vi "Hardware triggered acquisition - polling.vi"() -> ()   [LabVIEW 2015]
uses:
  SubVIs/Parameters Get & Set/Get Parameters/Get NumberOfQueuedFrames.vi
  SubVIs/Parameters Get & Set/Set Parameters/Set ExposureTime_us.vi
  SubVIs/Parameters Get & Set/Set Parameters/Set FramesPerTrigger_zeroForUnlimited.vi
  SubVIs/Parameters Get & Set/Set Parameters/Set OperationMode.vi
  C:/code/Host/Installer/Scientific Camera Interfaces/LabVIEW/64_bit/Library_X64/Thorlabs.TSI.TLCameraInterfaces.dll
  64_bit/Library_X64/Thorlabs.TSI.TLCameraInterfaces.dll
  SubVIs/Parameters Get & Set/Set Parameters/Set Gain.vi
panel:
  in  "Gain":u32 max=1023
  in  "Exposure (ms)":u32=100
  in  "stop":bool
  out "Intensity Graph":u16[][](graph)
  out "FrameNumber":u32
  in  "Frames Per Trigger":u32=1
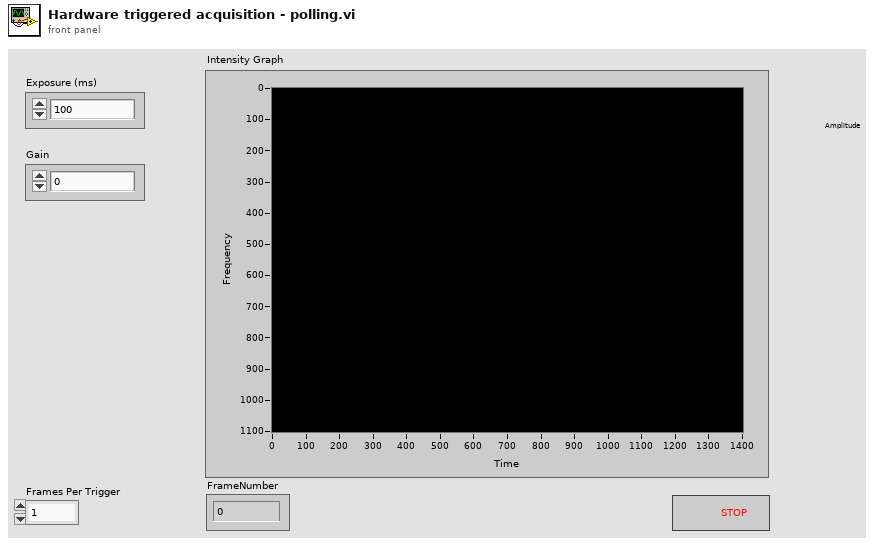
[diagram p1: front panel]
types:
  T1 = enum8{"Enabled", "Disabled", "Disabled and Grayed Out"}
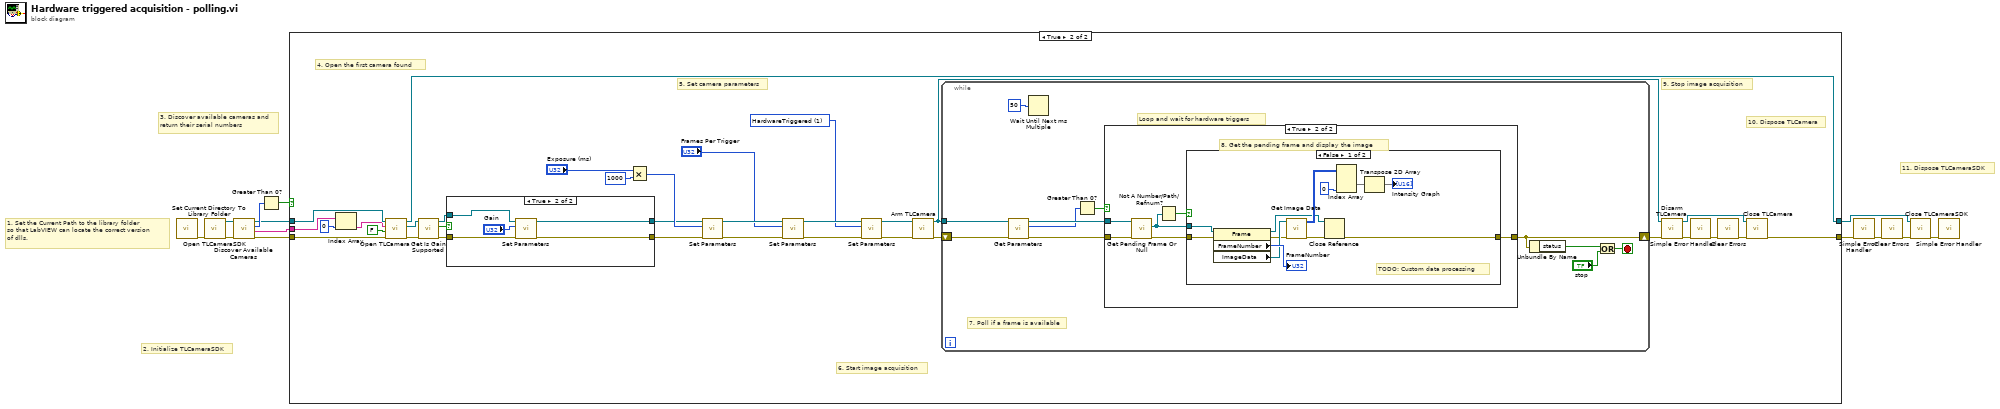
[diagram p0: block diagram]
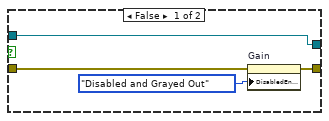
[diagram p3: hidden frame]
diagram:
  # "1. Set the Current Path to the library folder\nso that LabVIEW can locate the correct version\nof dlls."
  # "11. Dispose TLCameraSDK"
  # "3. Discover available cameras and\nreturn their serial numbers"
  # "2. Initialize TLCameraSDK"
  n1 = call "Set Current Directory To Library Folder.vi"() -> ("error out"=w7:errorcluster)  [unwired: 11 in]
  n2 = call "Open TLCameraSDK.vi"("error in (no error)"=w7) -> ("error out"=w6:errorcluster, "Thorlabs.TSI.TLCameraInterfaces.ITLCameraSDK"=w5:refnum<k24>)  [unwired: 9 in]
  n3 = call "Discover Available Cameras.vi"("error in (no error)"=w6, "Thorlabs.TSI.TLCameraInterfaces.ITLCameraSDK"=w5) -> ("error out"=w9:errorcluster, "Serial Numbers"=w11:string[], "Number of Cameras"=w13:i32, "Thorlabs.TSI.TLCameraInterfaces.ITLCameraSDK"=w10:refnum<k24>)  [unwired: 6 in]
  n4 = Greater Than 0?(x=w13) -> (x > 0?=w12:bool)
  n5 = case shown="True" w12 {
    tunnel: w11 -> [_ w47]
    tunnel: w10 -> [w14 w48]
    tunnel: w9 -> [w15 w38]
    tunnel: [w15 w35] -> w2
    tunnel: [w14 w43] -> w8
    frame False {
    }
    frame True {
      w23 = 1 items=["SoftwareTriggered", "HardwareTriggered", "Bulb", "Reserved1", "Reserved2"] ("OperationMode")
      # "10. Dispose TLCamera"
      # "9. Stop image acquisition"
      # "6. Start image acquisition"
      # "5. Set camera parameters"
      # "4. Open the first camera found"
      n6 = Index Array(array=w47, index=0) -> (element=w37:string)
      n7 = call "Open TLCamera.vi"("error in (no error)"=w38, "isDiagnosticsMessagesEnabled"=FALSE, "Camera serial number"=w37, "Thorlabs.TSI.TLCameraInterfaces.ITLCameraSDK"=w48) -> ("error out"=w19:errorcluster, "Thorlabs.TSI.TLCameraInterfaces.ITLCamera"=w18:refnum<k24>, "Thorlabs.TSI.TLCameraInterfaces.ITLCameraSDK"=w43:refnum<k24>)  [unwired: 5 in]
      n8 = call "Get Is Gain Supported.vi"("error in (no error)"=w19, "Thorlabs.TSI.TLCameraInterfaces.ITLCamera"=w18) -> ("error out"=w20:errorcluster, "Is Gain Supported?"=w22:bool, "Thorlabs.TSI.TLCameraInterfaces.ITLCamera"=w21:refnum<k24>)  [unwired: 7 in]
      n9 = case shown="True" w22 {
        tunnel: w21 -> [w50 w55]
        tunnel: w20 -> [w49 w57]
        tunnel: [w51 w56] -> w16
        tunnel: [w50 w54] -> w17
        frame False {
          n10 = property on="Gain" class="DigNum (strict)"(error in=w49, "DisabledEnum"=T1."Disabled and Grayed Out" ("Disabled")) -> (error out=w51:errorcluster)  [unwired: 1 in, 1 out]
        }
        frame True {
          n11 = call-poly "Set Parameters.vi"("error in (no error)"=w57, "Gain"="Gain", "Thorlabs.TSI.TLCameraInterfaces.ITLCamera"=w55) -> ("error out"=w56:errorcluster, "Thorlabs.TSI.TLCameraInterfaces.ITLCamera"=w54:refnum<k24>)  [unwired: 7 in]
        }
      }
      n12 = Multiply(x="Exposure (ms)", y=u32 1000) -> (x*y=w25:u32)
      n13 = call-poly "Set Parameters.vi"("error in (no error)"=w16, "ExposureTime_us"=w25, "Thorlabs.TSI.TLCameraInterfaces.ITLCamera"=w17) -> ("error out"=w28:errorcluster, "Thorlabs.TSI.TLCameraInterfaces.ITLCamera"=w31:refnum<k24>)  [unwired: 7 in]
      n14 = call-poly "Set Parameters.vi"("error in (no error)"=w28, "FramesPerTrigger_zeroForUnlimited"="Frames Per Trigger", "Thorlabs.TSI.TLCameraInterfaces.ITLCamera"=w31) -> ("error out"=w27:errorcluster, "Thorlabs.TSI.TLCameraInterfaces.ITLCamera"=w30:refnum<k24>)  [unwired: 7 in]
      n15 = call-poly "Set Parameters.vi"("error in (no error)"=w27, "OperationMode"=w23, "Thorlabs.TSI.TLCameraInterfaces.ITLCamera"=w30) -> ("error out"=w26:errorcluster, "Thorlabs.TSI.TLCameraInterfaces.ITLCamera"=w29:refnum<k24>)  [unwired: 7 in]
      n16 = call "Arm TLCamera.vi"("error in (no error)"=w26, "Thorlabs.TSI.TLCameraInterfaces.ITLCamera"=w29) -> ("error out"=w41:errorcluster, "Thorlabs.TSI.TLCameraInterfaces.ITLCamera"=w42:refnum<k24>)  [unwired: 8 in]
      n17 = while {
        tunnel: w42 -> [w62]
        shift-right: [w67] -> w36
        shift-left: w41 -> [w61]
        stop <- w64 stop-if-true
        # "Loop and wait for hardware triggers"
        # "7. Poll if a frame is available"
        n18 = call-poly "Get Parameters.vi"("error in (no error)"=w61, "Thorlabs.TSI.TLCameraInterfaces.ITLCamera"=w62) -> ("error out"=w60:errorcluster, "NumberOfQueuedFrames"=w59:i32, "Thorlabs.TSI.TLCameraInterfaces.ITLCamera"=w68:refnum<k24>)  [unwired: 7 in]
        n19 = Wait Until Next ms Multiple(millisecond multiple=u32 50) -> ()  [unwired: 1 out]
        n20 = Greater Than 0?(x=w59) -> (x > 0?=w58:bool)
        n21 = case shown="True" w58 {
          tunnel: w68 -> [_ w75]
          tunnel: [w69 w73] -> w67
          tunnel: w60 -> [w69 w72]
          frame False {
          }
          frame True {
            # "8. Get the pending frame and display the image"
            n22 = call "Get Pending Frame Or Null.vi"("error in (no error)"=w72, "Thorlabs.TSI.TLCameraInterfaces.ITLCamera"=w75) -> ("error out"=w70:errorcluster, "Thorlabs.TSI.TLCameraInterfaces.Frame"=w71:refnum<k24>)  [unwired: 7 in, 1 out]
            n23 = Not A Number/Path/Refnum?(number/path/refnum=w71) -> (NaN/Path/Refnum?=w74:bool)
            n24 = case shown="False" w74 {
              tunnel: w71 -> [w83 _]
              tunnel: w70 -> [w82 w88]
              tunnel: [w78 w88] -> w73
              frame False {
                # "TODO: Custom data processing"
                n25 = property class="Frame"(reference=w83, error in=w82) -> (reference out=w77:refnum<k24>, error out=w79:errorcluster, "FrameNumber"=→"FrameNumber":u32, "ImageData"=w80:refnum<k24>)
                n26 = call "Get Image Data.vi"("error in (no error)"=w79, "Thorlabs.TSI.ImageDataInterfaces.IImageData"=w80) -> ("error out"=w76:errorcluster, "Frame Data"=w84:u16[][][])  [unwired: 6 in, 2 out]
                n27 = Close Reference(reference=w77, error in (no error)=w76) -> (error out=w78:errorcluster)
                n28 = Index Array(array=w84, index (dim 2)=0 ("disabled index (col)")) -> (element=w86:u16[][])  [unwired: 2 in]
                n29 = Transpose 2D Array(2D array=w86) -> (transposed array=→"Intensity Graph":u16[][])
              }
              frame True {
              }
            }
          }
        }
        n30 = Unbundle By Name(w67) -> ("status"=w66:bool)
        n31 = Or(x=w66, y="stop") -> (x .or. y?=w64:bool)
      }
      n32 = call "Disarm TLCamera.vi"("error in (no error)"=w36, "Thorlabs.TSI.TLCameraInterfaces.ITLCamera"=w42) -> ("error out"=w34:errorcluster, "Thorlabs.TSI.TLCameraInterfaces.ITLCamera"=w44:refnum<k24>)  [unwired: 8 in]
      n33 = call <vilib>:"Simple Error Handler.vi"("error in (no error)"=w34) -> ("error out"=w33:errorcluster)  [unwired: 4 in, 4 out]
      n34 = call <vilib>:"Clear Errors.vi"("error in (no error)"=w33) -> ("error out"=w32:errorcluster)  [unwired: 5 in, 1 out]
      n35 = call "Close TLCamera.vi"("error in (no error)"=w32, "Thorlabs.TSI.TLCameraInterfaces.ITLCamera"=w44) -> ("error out"=w35:errorcluster)  [unwired: 9 in]
    }
  }
  n36 = call <vilib>:"Simple Error Handler.vi"("error in (no error)"=w2) -> ("error out"=w3:errorcluster)  [unwired: 4 in, 4 out]
  n37 = call <vilib>:"Clear Errors.vi"("error in (no error)"=w3) -> ("error out"=w1:errorcluster)  [unwired: 5 in, 1 out]
  n38 = call "Close TLCameraSDK.vi"("error in (no error)"=w1, "Thorlabs.TSI.TLCameraInterfaces.ITLCameraSDK"=w8) -> ("error out"=w4:errorcluster)  [unwired: 9 in]
  n39 = call <vilib>:"Simple Error Handler.vi"("error in (no error)"=w4) -> ()  [unwired: 4 in, 5 out]
